vi "Planta_Control_PI.vi"() -> ()   [LabVIEW 2012]
panel:
  out "control":dbl=1.0282304260481459
  in  "Entrada Deseada":dbl=3000.0
  in  "c(k-2)":dbl
  in  "c(k-1)":dbl
  in  "stop":bool
  in  "d1":dbl=2.0
  in  "d2":dbl=-2.0
  in  "d3":dbl
  in  "c1":dbl=0.0085
  in  "c2":dbl=-0.0085
  in  "c3":dbl
  out "Error":dbl=1076.0941417387598
  in  "b1":dbl=1.0
  in  "b2":dbl=-1.628
  in  "b3":dbl=0.6649
  in  "a1":dbl
  in  "a2":dbl=69.06
  in  "a3":dbl=0.001401
  in  "Periodo":i32=10
  in  "e(k-2)":dbl
  in  "e(k-1)":dbl
  in  "Y(k-2)":dbl
  in  "Y(k-1)":dbl
  out "Salida y(k)":dbl(graph)=1923.928295384087
  # "MODELO DE LA PLANTA"
  # "Z  +"
  # "Z^2  +"
  # "Gp(z) = --------------------------------------------------------"
  # "Z^2  +"
  # "Z  +"
  # "CONTROLADOR"
  # "Z  +"
  # "Z^2  +"
  # "Gp(z) = --------------------------------------------------------"
  # "Z^2  +"
  # "Z  +"
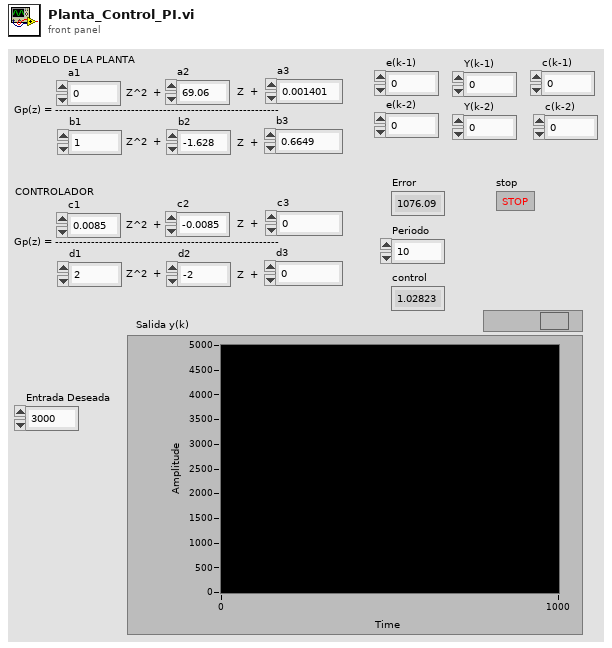
[diagram p1: front panel]
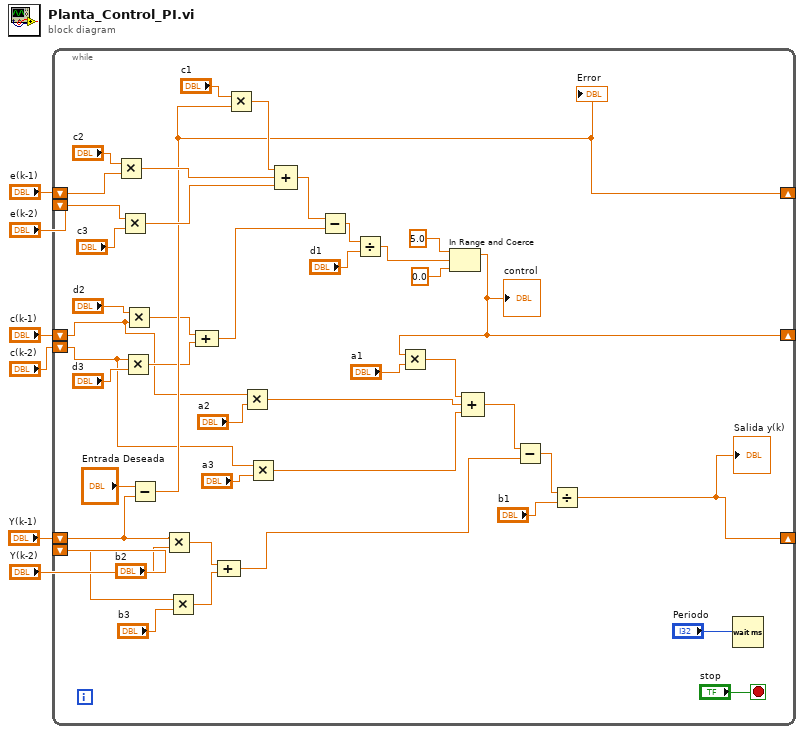
[diagram p0: block diagram]
diagram:
  n1 = while {
    shift-right: [w7] -> _
    shift-left: "Y(k-1)" -> [w35]
    shift-left: "Y(k-2)" -> [w44]
    shift-right: [w34] -> _
    shift-left: "e(k-1)" -> [w49]
    shift-left: "e(k-2)" -> [w48]
    shift-right: [w8] -> _
    shift-left: "c(k-1)" -> [w23]
    shift-left: "c(k-2)" -> [w21]
    stop <- "stop" stop-if-true
    n2 = Multiply(x="c2", y=w49) -> (x*y=w47:dbl)
    n3 = Multiply(x=w48, y="c3") -> (x*y=w46:dbl)
    n4 = Multiply(x=w21, y="d3") -> (x*y=w27:dbl)
    n5 = Multiply(x="d2", y=w23) -> (x*y=w28:dbl)
    n6 = Subtract(x="Entrada Deseada", y=w35) -> (x-y=w34:dbl)
    "Error" <- w34
    n7 = Multiply(x=w35, y="b2") -> (x*y=w42:dbl)
    n8 = Multiply(x=w44, y="b3") -> (x*y=w41:dbl)
    n9 = Compound Arithmetic op=ADD(w28, w27) -> (w26:dbl)
    n10 = Compound Arithmetic op=ADD(w42, w41) -> (w15:dbl)
    n11 = Multiply(x="c1", y=w34) -> (x*y=w38:dbl)
    n12 = Multiply(x=w23, y="a2") -> (x*y=w18:dbl)
    n13 = Multiply(x=w21, y="a3") -> (x*y=w17:dbl)
    n14 = Compound Arithmetic op=ADD(w38, w47, w46) -> (w40:dbl)
    n15 = Subtract(x=w40, y=w26) -> (x-y=w39:dbl)
    n16 = Divide(x=w39, y="d1") -> (x/y=w9:dbl)
    n17 = In Range and Coerce(upper limit=5.0, x=w9, lower limit=0.0) -> (coerced(x)=w8:dbl)  [unwired: 1 out]
    "control" <- w8
    n18 = Multiply(x=w8, y="a1") -> (x*y=w19:dbl)
    n19 = Compound Arithmetic op=ADD(w19, w18, w17) -> (w16:dbl)
    n20 = Subtract(x=w16, y=w15) -> (x-y=w14:dbl)
    n21 = Divide(x=w14, y="b1") -> (x/y=w7:dbl)
    "Salida y(k)" <- w7
    n22 = Wait (ms)(milliseconds to wait="Periodo") -> ()  [unwired: 1 out]
  }
